vi "find_repeat_parameters_3.vi"(8 "error in (no error)":errorcluster, 11 "String In":string="*RCL 0|1|2|3|4") -> (0 "error out":errorcluster, 3 "String Out":string="*RCL {0|1|2|3|4}")   [LabVIEW 2018]
uses:
  <vilib>/regexp/Match Regular Expression.xnode
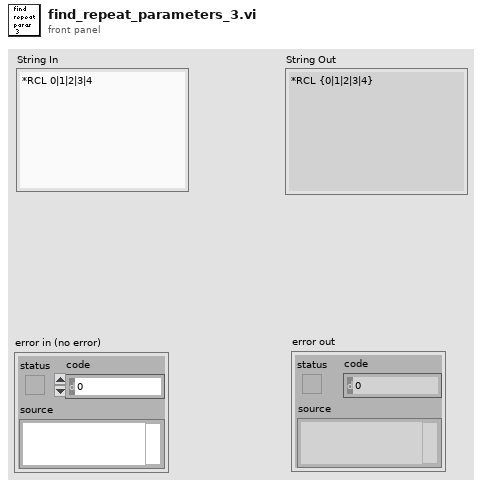
[diagram p1: front panel]
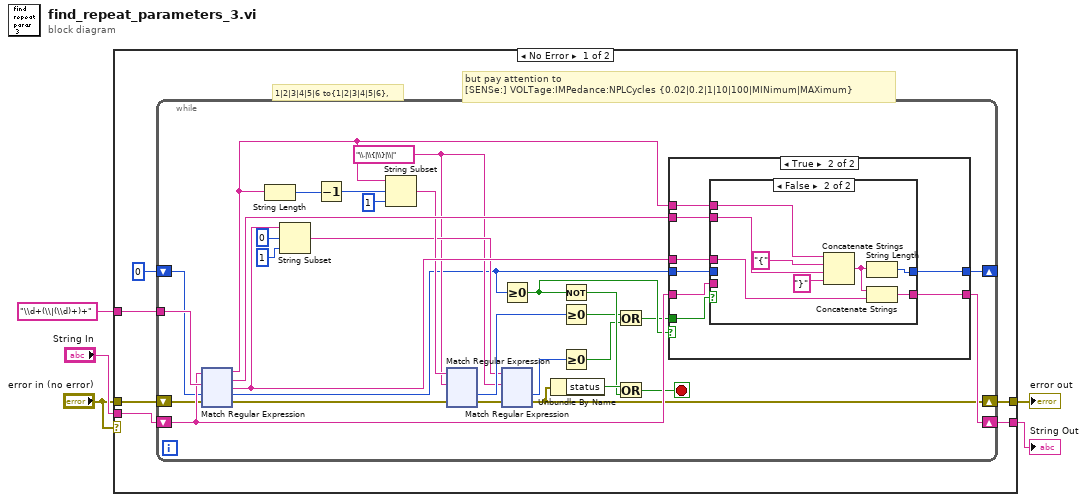
[diagram p0: block diagram]
diagram:
  n1 = case shown="No Error" "error in (no error)" {
    tunnel: "\\d+(\\|(\\d)+)+" ("regular expression") -> [w11 _]
    tunnel: "String In" -> [w8 w396]
    tunnel: [w10 w396] -> w3
    tunnel: "error in (no error)" -> [w7 w395]
    tunnel: [w9 w395] -> w2
    frame No Error {
      # "but pay attention to \n[SENSe:] VOLTage:IMPedance:NPLCycles {0.02|0.2|1|10|100|MINimum|MAXimum}"
      # "1|2|3|4|5|6 to{1|2|3|4|5|6},"
      n2 = while {
        tunnel: w11 -> [w41]
        shift-right: [w40] -> w10
        shift-left: w8 -> [w34]
        shift-right: [w18] -> w9
        shift-left: w7 -> [w33]
        shift-right: [w13] -> _
        shift-left: 0 ("offset (0)") -> [w28]
        stop <- w31 stop-if-true
        w20 = "\\.|\\{|\\}|\\|" ("regular expression")
        n3 = xnode "Match Regular Expression"("input string"=w34, "regular expression"=w41, "offset (0)"=w28, "error in"=w33) -> ("before match"=w37:string, "whole match"=w26:string, "after match"=w25:string, "offset past match"=w12:i32, "error out"=w27:errorcluster)  [unwired: 2 out]
        n4 = String Length(string=w37) -> (length=w38:i32)
        n5 = String Subset(string=w25, offset (0)=0, length (rest)=1 ("length (rest)")) -> (substring=w21:string)
        n6 = Decrement(x=w38) -> (x-1=w39:i32)
        n7 = String Subset(string=w37, offset (0)=w39, length (rest)=1 ("length (rest)")) -> (substring=w22:string)
        n8 = xnode "Match Regular Expression"("input string"=w22, "regular expression"=w20, "error in"=w27) -> ("offset past match"=w35:i32, "error out"=w19:errorcluster)  [unwired: 1 in, 5 out]
        n9 = Greater Or Equal To 0?(x=w12) -> (x >= 0?=w29:bool)
        n10 = xnode "Match Regular Expression"("input string"=w21, "regular expression"=w20, "error in"=w19) -> ("offset past match"=w17:i32, "error out"=w18:errorcluster)  [unwired: 1 in, 5 out]
        n11 = Unbundle By Name(w18) -> ("status"=w32:bool)
        n12 = Not(x=w29) -> (.not. x?=w30:bool)
        n13 = Greater Or Equal To 0?(x=w35) -> (x >= 0?=w15:bool)
        n14 = Greater Or Equal To 0?(x=w17) -> (x >= 0?=w16:bool)
        n15 = Or(x=w15, y=w16) -> (x .or. y?=w14:bool)
        n16 = Or(x=w32, y=w30) -> (x .or. y?=w31:bool)
        n17 = case shown="True" w29 {
          tunnel: w26 -> [_ w162]
          tunnel: [w154 w161] -> w40
          tunnel: w37 -> [_ w160]
          tunnel: w25 -> [_ w159]
          tunnel: w34 -> [w154 w157]
          tunnel: w14 -> [_ w158]
          tunnel: [w153 w156] -> w13
          tunnel: w12 -> [w153 w155]
          frame False {
          }
          frame True {
            n18 = case shown="False" w158 {
              tunnel: w162 -> [_ w171]
              tunnel: [w164 w167] -> w161
              tunnel: w160 -> [_ w172]
              tunnel: w159 -> [_ w168]
              tunnel: w157 -> [w164 _]
              tunnel: [w163 w165] -> w156
              tunnel: w155 -> [w163 _]
              frame True {
              }
              frame False {
                n19 = Concatenate Strings(w172, "{" ("string"), w171, "}" ("string")) -> (w166:string)
                n20 = String Length(string=w166) -> (length=w165:i32)
                n21 = Concatenate Strings(w166, w168) -> (w167:string)
              }
            }
          }
        }
      }
    }
    frame Error {
    }
  }
  "String Out" <- w3
  "error out" <- w2
